vi "Read Data Bits.vi"(8 "error in (no error)":errorcluster, 11 "ASCII Data Unit in":refnum<class "ASCII Data Unit.lvclass">) -> (0 "error out":errorcluster, 2 "data bits":u16=7, 3 "ASCII Data Unit out":refnum<class "ASCII Data Unit.lvclass">)   [LabVIEW 2012, in "ASCII Data Unit.lvclass"]
doc: "Acts as a constant, and provides a way for the serial slave to properly configure the serial interface. 7 bits in this case."
uses:
  ASCII Data Unit.lvclass
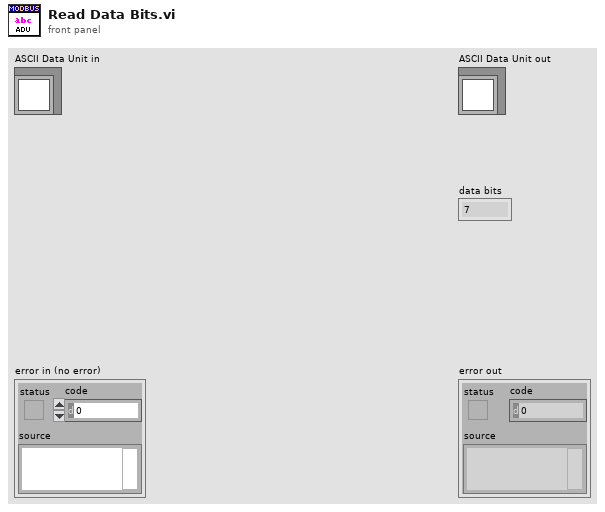
[diagram p1: front panel]
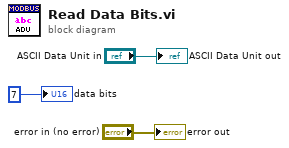
[diagram p0: block diagram]
diagram:
  "error out" <- "error in (no error)"
  "ASCII Data Unit out" <- "ASCII Data Unit in"
  "data bits" <- u16 7 ("data bits")
